vi "oax_gsPlay Sound+.vi"(0 "Array":i16[](array[numeric]), 2 "sound format":T1) -> ()   [LabVIEW 2017]
uses:
  <vilib>/addons/Sound and Vibration/Order Analysis/Example Support/Demo VI/subVIs/oax_gsSound Format+.ctl
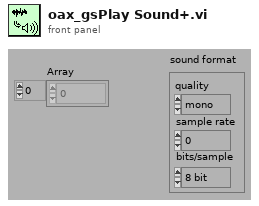
[diagram p1: front panel]
types:
  T1 = typedef "oax_gsSound Format+.ctl" = cluster{"quality":enum16{"mono", "stereo"}, "sample rate":u32, "bits/sample":enum16{"8 bit", "16 bit"}}
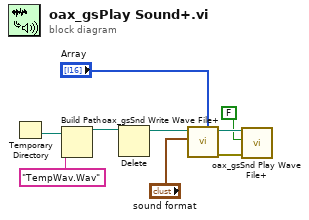
[diagram p0: block diagram]
diagram:
  n1 = Temporary Directory() -> (w7:path)
  n2 = Build Path(base path=w7, name or relative path="TempWav.Wav") -> (appended path=w2:path)
  n3 = Delete(path (use dialog)=w2) -> (deleted path=w1:path)  [unwired: 4 in, 2 out]
  n4 = call <vilib>:"oax_gsSnd Write Wave File+.vi"("mono 16-bit"="Array", "sound format"="sound format", "wave file path"=w1) -> ("error out"=w3:errorcluster, "wave file path out"=w5:path)  [unwired: 7 in]
  n5 = call <vilib>:"oax_gsSnd Play Wave File+.vi"("error in (no error)"=w3, "wait until finish (T)"=FALSE, "wave file path in"=w5) -> ()  [unwired: 7 in, 2 out]
